vi "picoquant_get_count_rates.vi"(8 "error in (no error)":errorcluster, 11 "hydraharp in":refnum<class "hydraharp.lvclass">) -> (0 "error out":errorcluster, 2 "count_rates":T1, 3 "hydraharp out":refnum<class "hydraharp.lvclass">)   [LabVIEW 2015, in "hydraharp.lvclass"]
uses:
  hydraharp.lvclass
  hydraharp_count_rates.ctl
  hydraharp.lvclass/hydraharp.ctl
  hhlib.dll
panel:
  out "get_counts_error":i32
  out "sync_error":i32
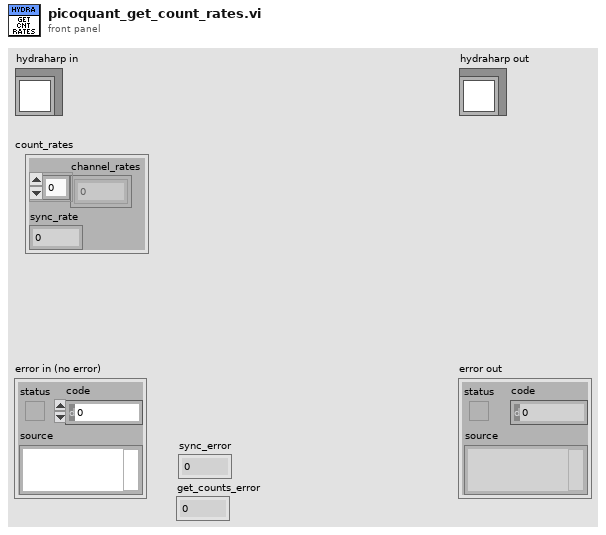
[diagram p1: front panel]
types:
  T1 = typedef "hydraharp_count_rates.ctl" = cluster{"channel_rates":i32[], "sync_rate":i32}
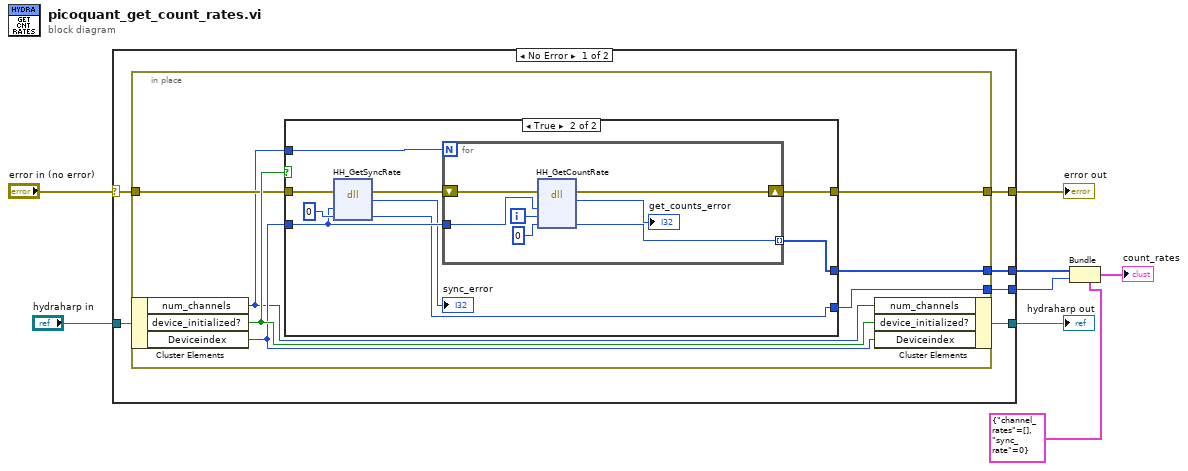
[diagram p0: block diagram]
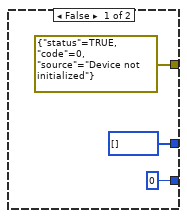
[diagram p2: hidden frame]
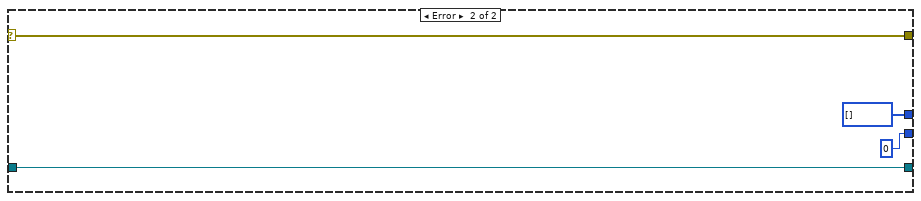
[diagram p3: hidden frame]
diagram:
  n1 = case shown="No Error" "error in (no error)" {
    selector: "error in (no error)" -> [w13 w44]
    tunnel: [w12 w44] -> w2
    tunnel: [w10 w43] -> w6
    tunnel: "hydraharp in" -> [w14 w43]
    tunnel: [w11 i32[] []] -> w5
    tunnel: [w9 0 ("rate")] -> w4
    frame No Error {
      n2 = in-place {
        in-place-border: w13 -> [w20]
        in-place-border: [w18] -> w12
        in-place-border: [w17] -> w11
        in-place-border: [w16] -> w9
        n3 = in-place-cluster #1(w14) -> ("num_channels"=w15:i32, "device_initialized?"=w21:bool, "Deviceindex"=w19:i32)
        n4 = case shown="True" w21 {
          tunnel: w20 -> [_ w33]
          tunnel: w19 -> [_ w30]
          tunnel: [i32[] [] w29] -> w17
          tunnel: [0 ("rate") w28] -> w16
          tunnel: [errorcluster {"status"=TRUE, "code"=0, "source"="Device not initialized"} ("error out") w27] -> w18
          tunnel: w15 -> [_ w25]
          frame False {
          }
          frame True {
            n5 = dll-call lib="hhlib.dll" fn="HH_GetSyncRate"(error in=w33, "devidx"=w30, "rate"=0) -> (error out=w31:errorcluster, →"sync_error":i32, "rate"=w28:i32)  [unwired: 3 in, 1 out]
            n6 = for {
              N: w25 -> [_]
              shift-right: [w39] -> w27
              shift-left: w31 -> [w40]
              tunnel: w30 -> [w38]
              tunnel: [w35] -> w29 mode=indexing
              i -> [w37]
              n7 = dll-call lib="hhlib.dll" fn="HH_GetCountRate"(error in=w40, "devidx"=w38, "channel"=w37, "rate"=0) -> (error out=w39:errorcluster, →"get_counts_error":i32, "rate"=w35:i32)  [unwired: 4 in, 1 out]
            }
          }
        }
        n8 = in-place-cluster #1("num_channels"=w15, "device_initialized?"=w21, "Deviceindex"=w19) -> (w10:refnum<class "hydraharp.lvclass">)
      }
    }
    frame Error {
    }
  }
  "error out" <- w2
  "hydraharp out" <- w6
  n9 = Bundle(cluster=T1 {"channel_rates"=[], "sync_rate"=0} ("output cluster"), "channel_rates"=w5, "sync_rate"=w4) -> (→"count_rates":T1)
